vi "LVRT Serial Read.vi"(8 "error in (no error)":errorcluster, 9 "Timeout (ms) (-1: no timeout)":i32=-1, 10 "Bytes to Read":u32, 11 "FPGA Main Ref":T1) -> (0 "error out":errorcluster, 2 "Read: Char":u8, 3 "FPGA Main Ref Out":T1)   [LabVIEW 2014]
uses:
  Controls/FPGA Reference.ctl
  <vilib>/rvi/errors/niLvFpgaAdjustHostInterfaceError.vi
  <vilib>/rvi/interface/nirviReadWriteControl/nirviReadWriteControl.xnode
  <vilib>/rvi/interface/Simulation/niFpgaSimulationCallBeginRW.vi
  NiFpgaLv.dll
panel:
  out "Bytes read so far":u32
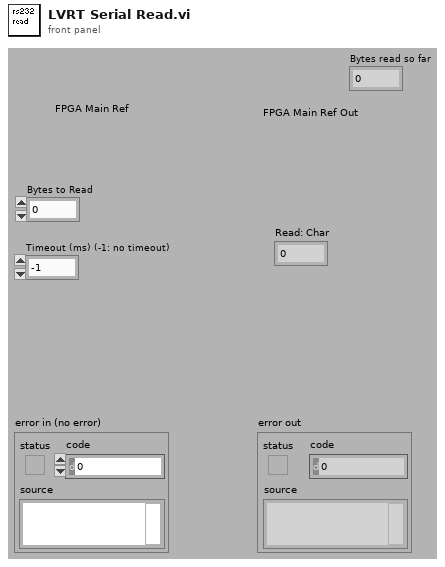
[diagram p1: front panel]
types:
  T1 = typedef "FPGA Reference.ctl" = refnum<k20>
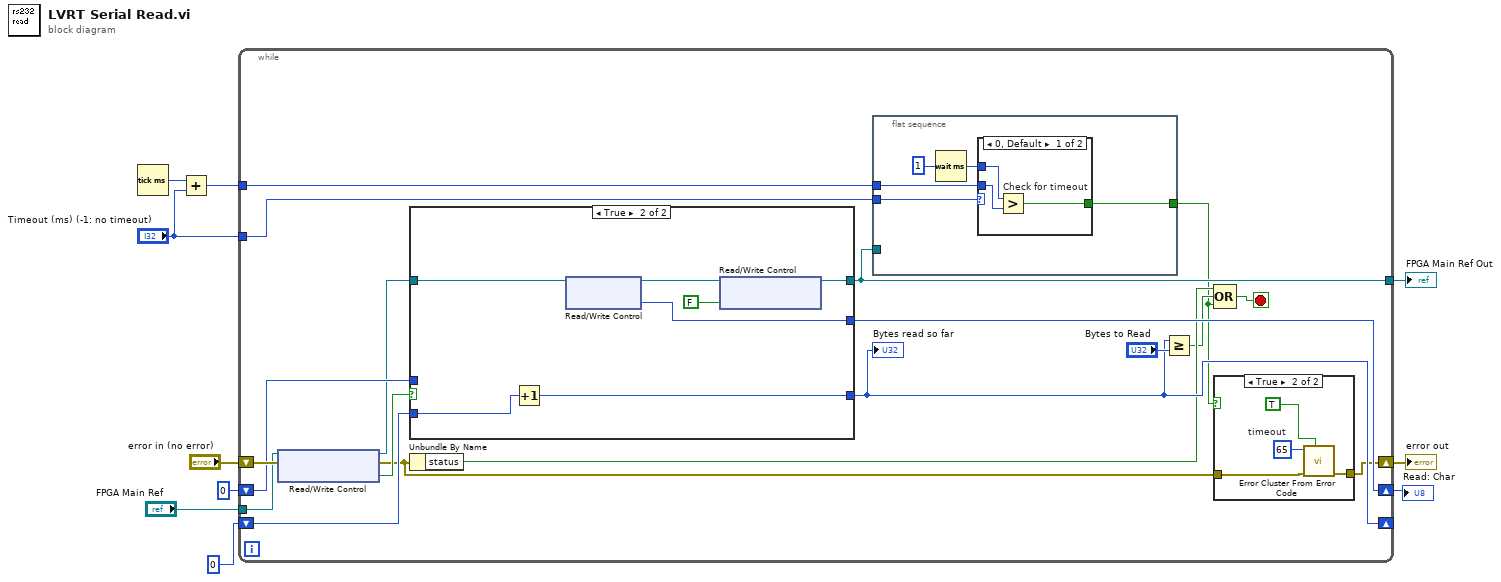
[diagram p0: block diagram]
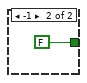
[diagram p3: hidden frame]
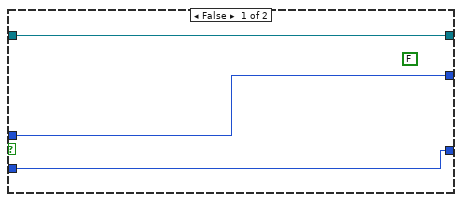
[diagram p4: hidden frame]
diagram:
  n1 = Tick Count (ms)() -> (millisecond timer value=w5:u32)
  n2 = Add(x=w5, y="Timeout (ms) (-1: no timeout)") -> (x+y=w3:u32)
  n3 = while {
    tunnel: "FPGA Main Ref" -> [w22]
    tunnel: [w20] -> w7
    shift-right: [w19] -> _
    shift-left: u32 0 -> [w26]
    shift-right: [w24] -> w1
    shift-left: u8 0 ("Read: Char") -> [w25]
    shift-right: [w12] -> w9
    shift-left: "error in (no error)" -> [w28]
    tunnel: "Timeout (ms) (-1: no timeout)" -> [w15]
    tunnel: w3 -> [w14]
    stop <- w16 stop-if-true
    n4 = xnode "Read/Write Control"("FPGA VI Reference In"=w22, "error in"=w28) -> ("FPGA VI Reference Out"=w21:T1, "error out"=w13:errorcluster, "Read: New Data"=w27:bool)
    n5 = case shown="True" w27 {
      tunnel: [w45 w52] -> w19
      tunnel: w26 -> [w45 w51]
      tunnel: w25 -> [w44 _]
      tunnel: [w44 w46] -> w24
      tunnel: w21 -> [w43 w50]
      tunnel: [w43 w48] -> w20
      frame False {
        (unwired) FALSE
      }
      frame True {
        n6 = Increment(x=w51) -> (x+1=w52:u32)
        n7 = xnode "Read/Write Control"("FPGA VI Reference In"=w50) -> ("FPGA VI Reference Out"=w49:T1, "Read: Char"=w46:u8)  [unwired: 1 in, 1 out]
        n8 = xnode "Read/Write Control"("FPGA VI Reference In"=w49, "Read: New Data"=FALSE ("Data Read")) -> ("FPGA VI Reference Out"=w48:T1)  [unwired: 1 in, 1 out]
      }
    }
    "Bytes read so far" <- w19
    n9 = Unbundle By Name(w13) -> ("status"=w18:bool)
    n10 = flat-sequence {
      tunnel: w20 -> [_]
      tunnel: [w37] -> w11
      tunnel: w15 -> [w36]
      tunnel: w14 -> [w35]
      frame #0 {
        n11 = Wait (ms)(milliseconds to wait=u32 1) -> (millisecond timer value=w34:u32)
        n12 = case shown="0, Default" w36 {
          tunnel: [w39 FALSE] -> w37
          tunnel: w35 -> [w40 _]
          tunnel: w34 -> [w41 _]
          frame 0, Default {
            n13 = Greater? "Check for timeout"(x=w41, y=w40) -> (0:w39:bool)
          }
          frame -1 {
          }
        }
      }
    }
    n14 = Greater Or Equal?(x=w19, y="Bytes to Read") -> (x >= y?=w17:bool)
    n15 = Compound Arithmetic op=OR(w18, w17, w11) -> (w16:bool)
    n16 = case shown="True" w11 {
      tunnel: w13 -> [w29 w33]
      tunnel: [w29 w32] -> w12
      frame False {
      }
      frame True {
        w31 = 65  # timeout
        n17 = call <vilib>:"Error Cluster From Error Code.vi"("show call chain? (False)"=TRUE, "error in (no error)"=w33, "error code (0)"=w31) -> ("error out"=w32:errorcluster)  [unwired: 6 out]
      }
    }
  }
  "error out" <- w9
  "FPGA Main Ref Out" <- w7
  "Read: Char" <- w1
